vi "Square Wave Out.vi"(8 "Frequency":u32, 9 "Duty Cycle":u32, 11 "FPGA I/O":refnum<k21>="Connector0/DIO0") -> ()   [LabVIEW 2010]
uses:
  <vilib>/eio/EIONode/EIONode.xnode
  <vilib>/rvi/eio/nirviEIOImplementation/nirviEIOImplementation.xnode
  <vilib>/rvi/eio/common/nirviEmuClasses.ctl
  <vilib>/rvi/eio/common/nirviEmuTemplateMethod_noerrors.vi
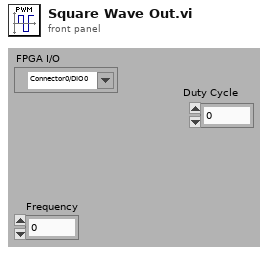
[diagram p1: front panel]
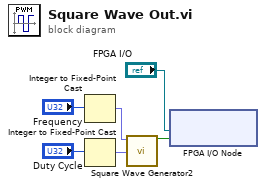
[diagram p0: block diagram]
diagram:
  n1 = Integer to Fixed-Point Cast(integer="Frequency") -> (fixed-point=w5:fxp<+,32,0>)  [unwired: 1 in]
  n2 = Integer to Fixed-Point Cast(integer="Duty Cycle") -> (fixed-point=w3:fxp<+,32,0>)  [unwired: 1 in]
  n3 = call "Square Wave Generator2"("frequency (periods/tick)"=w5, "duty cycle (periods)"=w3) -> ("square wave out"=w6:bool)  [unwired: 13 in]
  n4 = xnode "FPGA I/O Node"("I/O Item"=w6, "FPGA I/O In"="FPGA I/O") -> ()  [unwired: 1 out]
